vi "Type.FG.vi"(7 "Action":T1, 8 "error in (no error)":errorcluster, 10 "Type":T2, 11 "Device Item Ref in":T3 format="%.0x") -> (0 "error out":errorcluster, 2 "Type":T2, 3 "Device Item Ref out":T3=18446744073709551615 format="%.0x")   [LabVIEW 2015, in "Diagnostics Addon System Explorer.lvlib"]
uses:
  Diagnostics Addon System Explorer.lvlib
  <vilib>/NI Veristand/Custom Device API/Custom Device Item Ref.ctl
  Shared/Types/Type.ctl
  Types/FG.Action.ctl
  <vilib>/NI Veristand/Custom Device API/Get Item Property (U32).vi
  <vilib>/NI/NI VeriStand Advanced SysDef API/_SubVIs/SysDef.Property.Set.U32.vi
  Shared/SubVIs/Constants.vi
  Shared/Diagnostics Addon Shared.lvlib
  <vilib>/NI Veristand/Custom Device API/Custom Device API.lvlib
  <vilib>/NI/NI VeriStand Advanced SysDef API/SysDef API/Advanced System Definition.lvlib
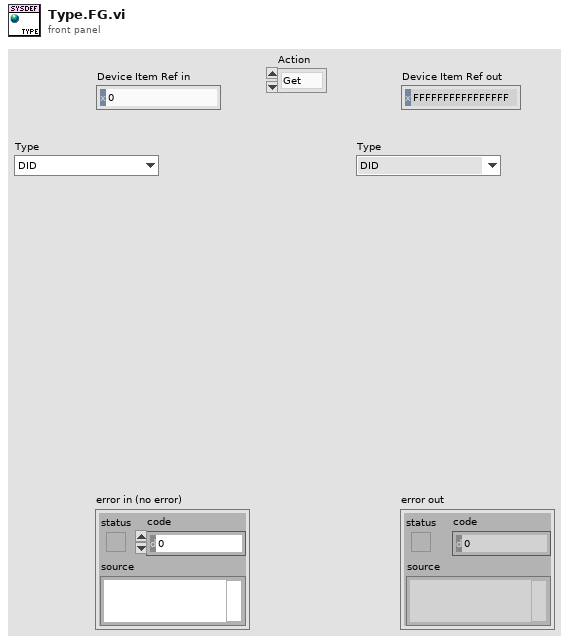
[diagram p1: front panel]
types:
  T1 = typedef "Diagnostics Addon System Explorer.lvlib/FG.Action.ctl" = enum16{"Get", "Set"}
  T2 = typedef "Diagnostics Addon Shared.lvlib/Type.ctl" = enum16{"DID", "CDID", "PID", "CPID", "Read Memory", "Write Memory", "DTC Control", "IO Cmd", "IO Resp", "Routine Start Cmd", "Routine Start Resp", "Routine Request Cmd", "Routine Request Resp", "Routine Stop Cmd", "Routine Stop Resp", "UserDefined Cmd", "UserDefined Rsp"}
  T3 = typedef "Custom Device API.lvlib/Custom Device Item Ref.ctl" = u64
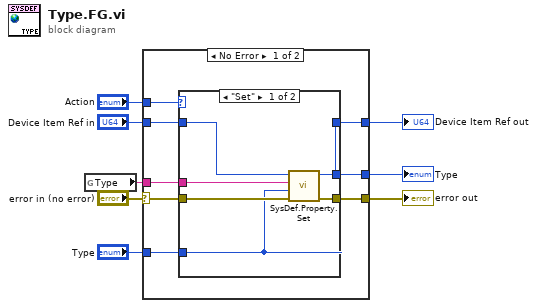
[diagram p0: block diagram]
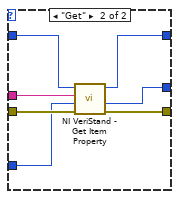
[diagram p2: hidden frame]
diagram:
  n1 = global read "Constants.vi" "Type"() -> (w3:string)
  n2 = case shown="No Error" "error in (no error)" {
    selector: "error in (no error)" -> [w16 w30]
    tunnel: "Device Item Ref in" -> [w15 w31]
    tunnel: [w14 w31] -> w5
    tunnel: [w13 w30] -> w6
    tunnel: [w12 _] -> w4
    tunnel: w3 -> [w11 _]
    tunnel: "Type" -> [w10 _]
    tunnel: "Action" -> [w9 _]
    frame No Error {
      n3 = case shown="\"Set\"" w9 {
        tunnel: w16 -> [w22 w29]
        tunnel: w15 -> [w19 w28]
        tunnel: [w18 w27] -> w14
        tunnel: [w21 w24] -> w13
        tunnel: [w17 w23] -> w12
        tunnel: w11 -> [w20 w26]
        tunnel: w10 -> [w17 w25]
        frame "Set" {
          n4 = call-poly <vilib>:"SysDef.Property.Set.vi"("error in (no error)"=w22, "Value"=w17, "Property Name"=w20, "nodeID"=w19) -> ("error out"=w21:errorcluster, "nodeID out"=w18:u64)  [unwired: 6 in]
        }
        frame "Get" {
          n5 = call-poly <vilib>:"NI VeriStand - Get Item Property.vi"("error in (no error)"=w29, "Default Value"=w25, "Property Name"=w26, "Item Ref in"=w28) -> ("error out"=w24:errorcluster, "Value"=w23:u32, "Item Ref out"=w27:T3)  [unwired: 4 in, 1 out]
        }
      }
    }
    frame Error {
    }
  }
  "error out" <- w6
  "Device Item Ref out" <- w5
  "Type" <- w4
